vi "2017 Washer Backsplash Tester Main.vi"() -> ()   [LabVIEW 2016]
uses:
  controls/states.ctl
  controls/Stop Button.ctl
  controls/Test Results.ctl
  controls/Error_Command.ctl
  C:/Program Files (x86)/National Instruments/LabVIEW 2016/examples/Design Patterns/Queued Message Handler/support/QMH Fundamentals - Message Cluster.ctl
  C:/Automation/DLLs/PC Dot Net/GeaCommunication.dll
  Common/LabVIEW GEA2 Toolkit/LabVIEW_GEA2_Toolkit.lvlibp
panel:
  out "Test Results out":T1
  in  "Stop Button":T2
  out "State":T3
  in  "Barcode Scan":string
  out "Error Out":errorcluster
  in  "Error In":errorcluster
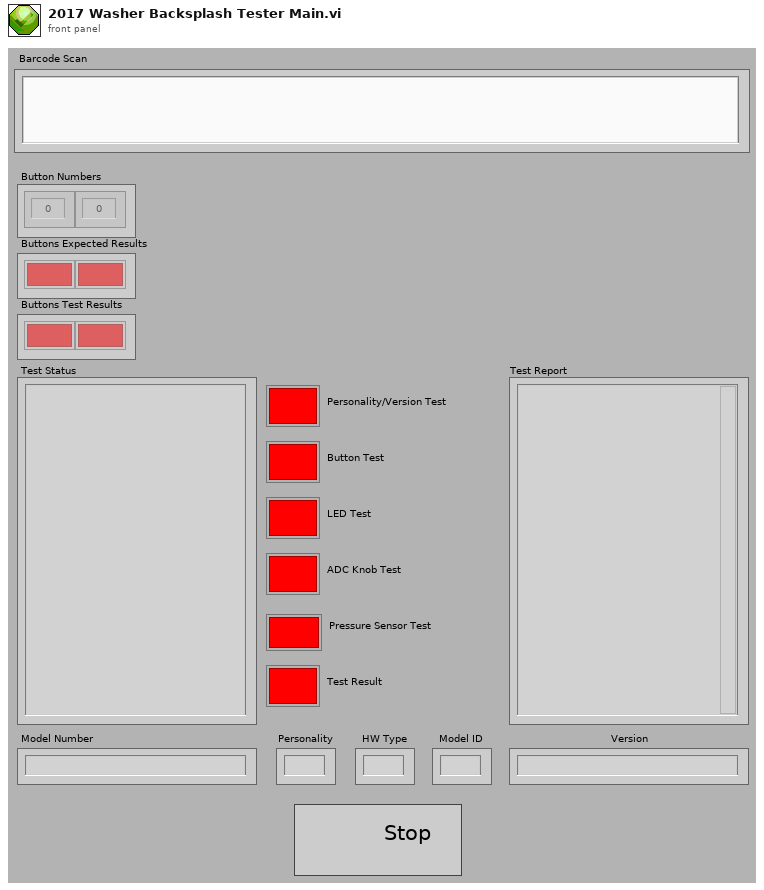
[diagram p1: front panel]
types:
  T1 = cluster{"Test Status":string, "Personality/Version Test ":bool, "Test Report":string, "Model Number":string, "Button Numbers":i32[], "Buttons Test Results":bool[], "Buttons Expected Results":bool[], "Model ID":string, "Personality":string, "HW Type":string, "Version":string, "Button Test":bool, "LED Test":bool, "ADC Knob Test":bool, "Pressure Sensor Test":bool, "Test Result":bool}
  T2 = typedef "Stop Button.ctl" = bool
  T3 = typedef "states.ctl" = enum16{"Wait for Barcode Scan", "Confirm Board Setup", "Initialization", "Perosnality Test", "Button Test", "LED Test", "ADC Knob Test", "Pressure Sensor Test", "Test Complete", "Log Results", "Re-Init Test", "Shutdown"}
  T4 = typedef "QMH Fundamentals - Message Cluster.ctl" = cluster{"Message":string, "Message Data":variant}
  T5 = typedef "Error_Command.ctl" = enum16{"Initialize", "Handle Errors", "Report Errors"}
  T6 = typedef "Test Results.ctl" = cluster{"Test Status":string, "Personality/Version Test ":bool, "Test Report":string, "Model Number":string, "Button Numbers":i32[], "Buttons Test Results":bool[], "Buttons Expected Results":bool[], "Model ID":string, "Personality":string, "HW Type":string, "Version":string, "Button Test":bool, "LED Test":bool, "ADC Knob Test":bool, "Pressure Sensor Test":bool, "Test Result":bool}
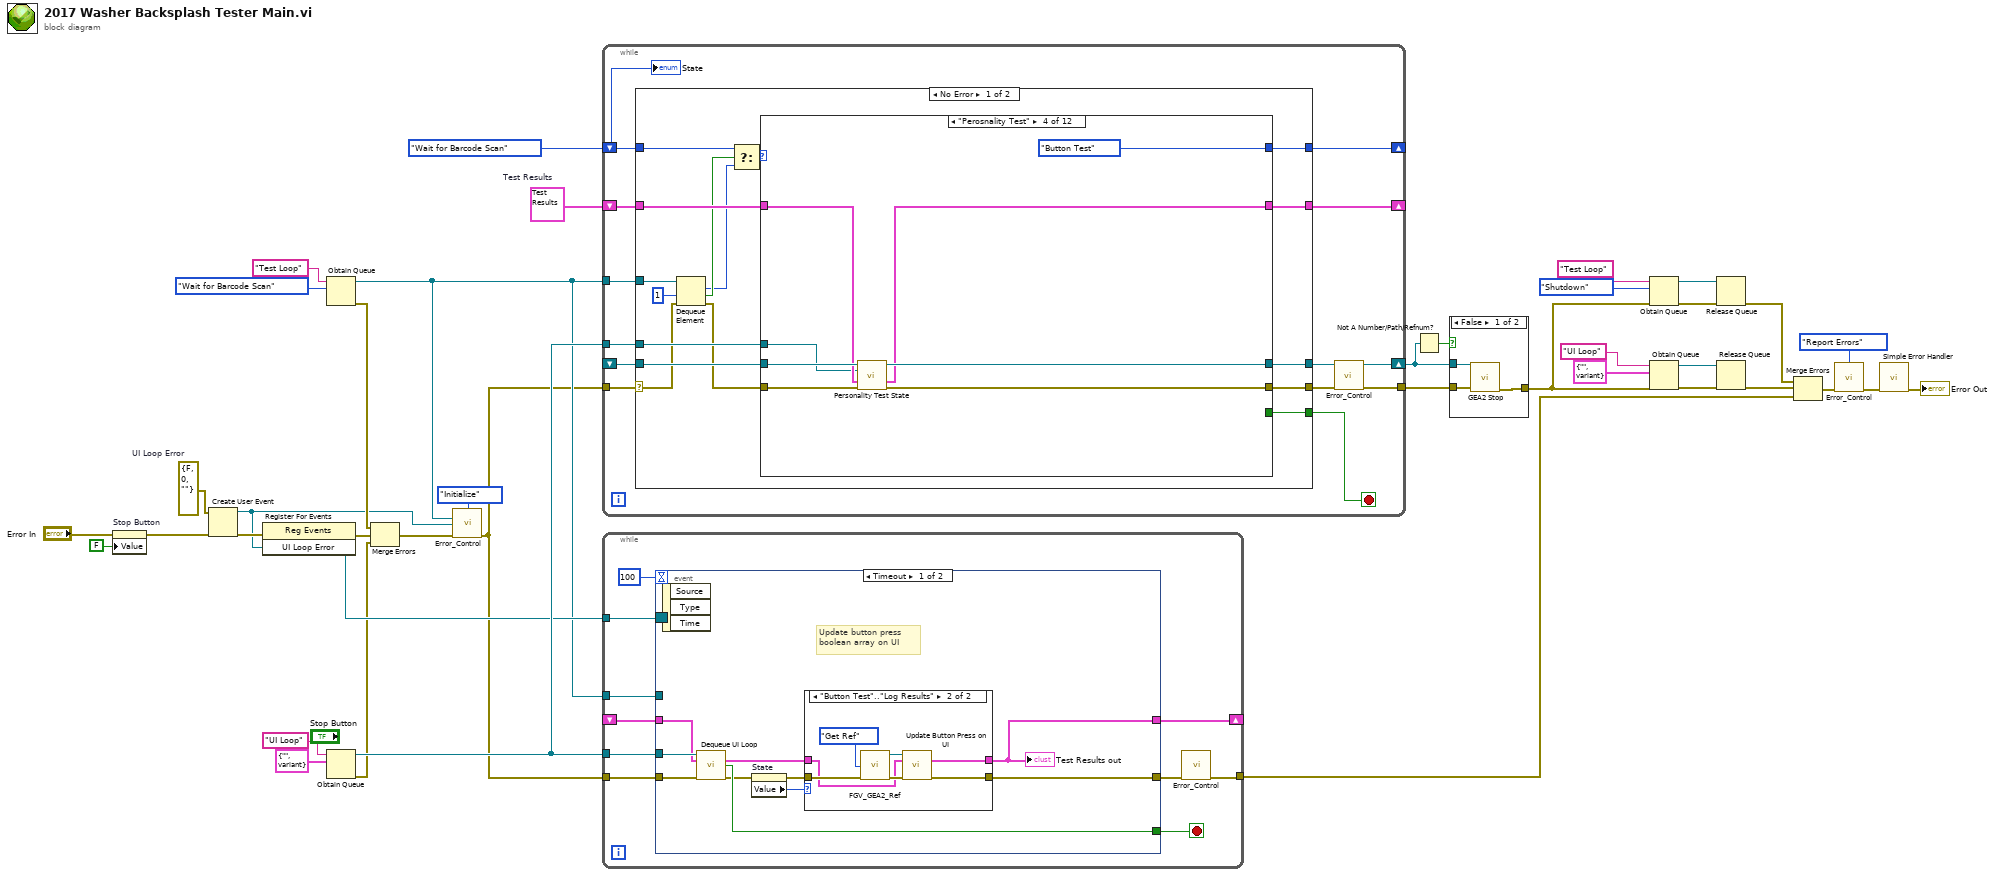
[diagram p0: block diagram]
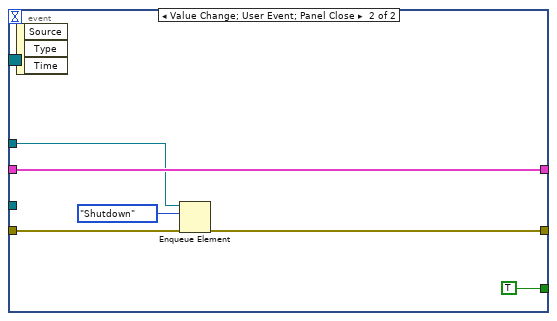
[diagram p4: hidden frame]
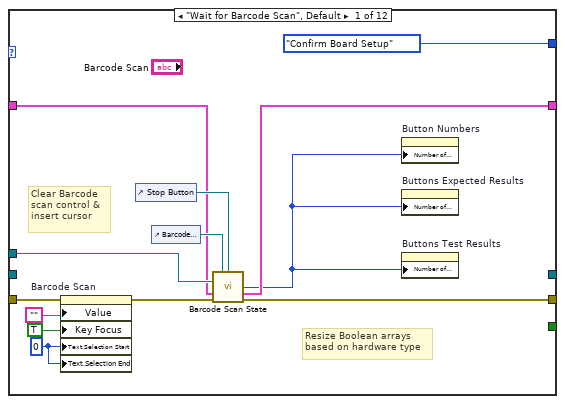
[diagram p5: hidden frame]
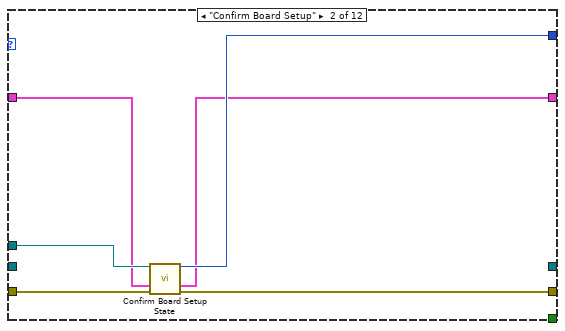
[diagram p6: hidden frame]
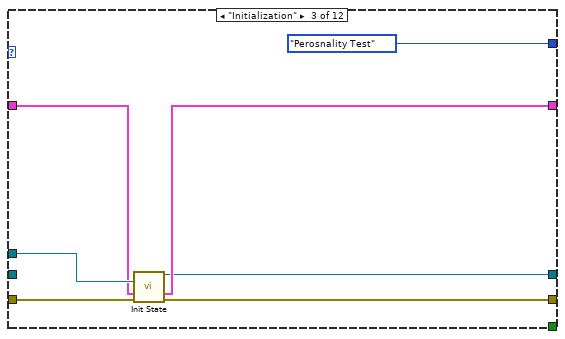
[diagram p7: hidden frame]
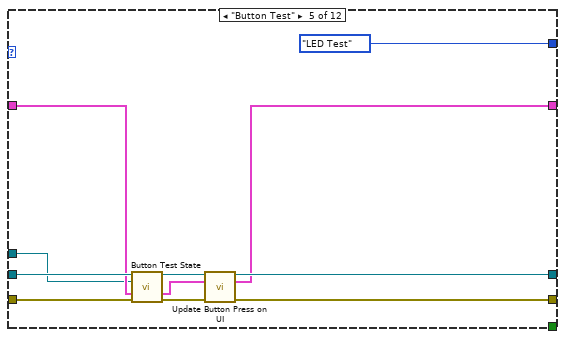
[diagram p8: hidden frame]
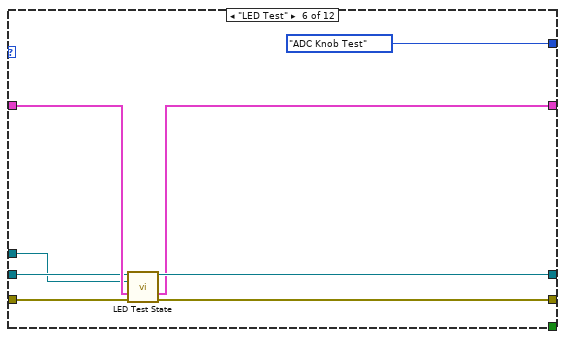
[diagram p9: hidden frame]
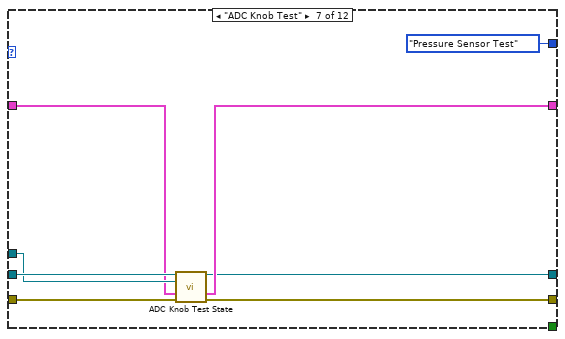
[diagram p10: hidden frame]
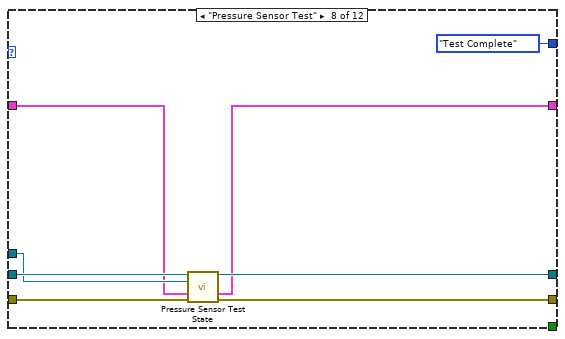
[diagram p11: hidden frame]
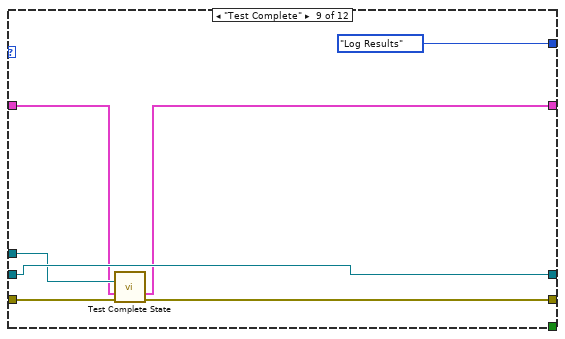
[diagram p12: hidden frame]
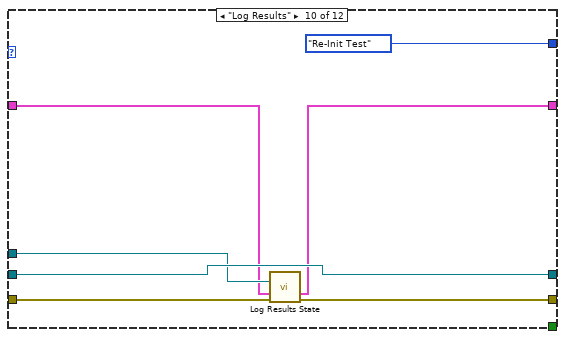
[diagram p13: hidden frame]
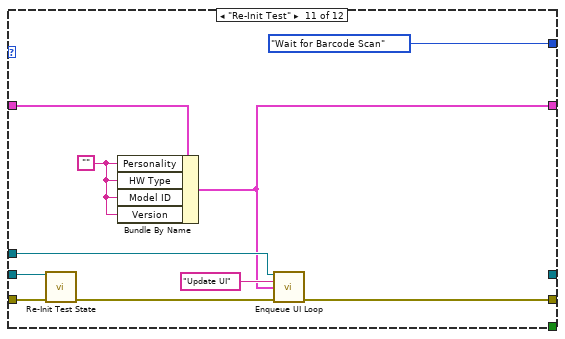
[diagram p14: hidden frame]
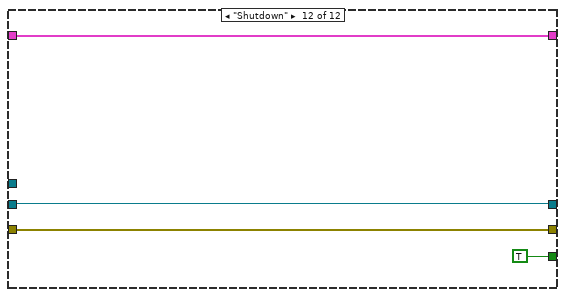
[diagram p15: hidden frame]
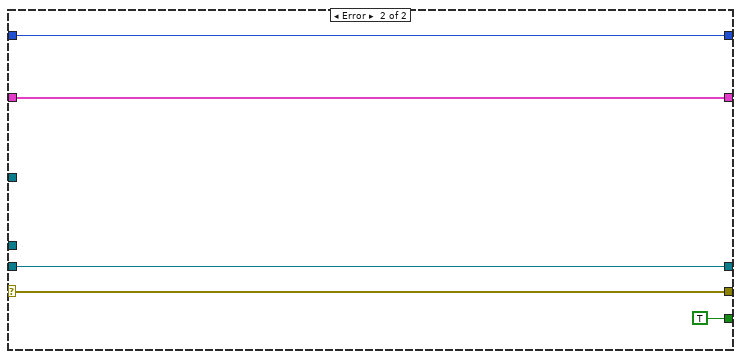
[diagram p16: hidden frame]
diagram:
  w14 = errorcluster {"status"=FALSE, "code"=0, "source"=""}  # UI Loop Error
  w39 = T6 {"Test Status"="", "Personality/Version Test "=FALSE, "Test Report"="", "Model Number"="", "Button Numbers"=[], "Buttons Test Results"=[], "Buttons Expected Results"=[], "Model ID"="", "Personality"="", "HW Type"="", "Version"="", "Button Test"=FALSE, "LED Test"=FALSE, "ADC Knob Test"=FALSE, "Pressure Sensor Test"=FALSE, "Test Result"=FALSE}  # Test Results
  n1 = property on="Stop Button" class="Bool (strict)"(error in="Error In", "Value"=FALSE ("Stop Button")) -> (error out=w13:errorcluster)  [unwired: 1 in, 1 out]
  n2 = Create User Event(user event datatype=w14, error in=w13) -> (user event=w8:refnum<user-event>, error out=w15:errorcluster)
  n3 = register-events(error in=w15, w8) -> (reference out=w11:refnum<event-registration>, error out=w3:errorcluster)  [unwired: 1 in]
  n4 = Obtain Queue(name (unnamed)="Test Loop", element data type=states."Wait for Barcode Scan" ("Enum")) -> (queue out=w9:refnum<queue>, error out=w12:errorcluster)  [unwired: 3 in, 1 out]
  n5 = Obtain Queue(name (unnamed)="UI Loop", element data type=T4 {"Message"="", "Message Data"=variant} ("Message Cluster")) -> (queue out=w38:refnum<queue>, error out=w2:errorcluster)  [unwired: 3 in, 1 out]
  n6 = Merge Errors(w12, w3, w2) -> (w10:errorcluster)
  n7 = call "Error_Control.vi"("Command (Handle Errors)"=Error_Command."Initialize", "Test Loop"=w9, "UI Loop Error"=w8, "Error In"=w10) -> ("Error Out"=w7:errorcluster)  [unwired: 11 in]
  n8 = while {
    shift-right: [w51] -> _
    shift-left: w39 -> [w52]
    shift-right: [w50] -> _
    shift-left: states."Wait for Barcode Scan" ("Enum") -> [w46]
    tunnel: [w42] -> w33
    shift-right: [w49] -> w27
    shift-left: _ -> [w48]
    tunnel: w38 -> [w47]
    tunnel: w9 -> [w45]
    tunnel: w7 -> [w41]
    stop <- w44 stop-if-true
    n9 = case shown="No Error" w41 {
      selector: w41 -> [w54 w169]
      tunnel: w46 -> [w58 w168]
      tunnel: w52 -> [w68 w167]
      tunnel: [w67 w167] -> w51
      tunnel: [w66 w168] -> w50
      tunnel: [w65 w169] -> w43
      tunnel: [w64 w170] -> w49
      tunnel: w48 -> [w63 w170]
      tunnel: w47 -> [w62 _]
      tunnel: w45 -> [w61 _]
      tunnel: [w56 TRUE] -> w44
      frame No Error {
        n10 = Dequeue Element(queue=w61, timeout in ms (-1)=1, error in (no error)=w54) -> (element=w57:T3, timed out?=w59:bool, error out=w53:errorcluster)  [unwired: 1 out]
        n11 = Select(t=w58, s=w59, f=w57) -> (s? t:f=w60:T3)
        n12 = case shown="\"Perosnality Test\"" w60 {
          tunnel: w68 -> [w74 w83 w88 w100 w111 w120 w124 w131 w140 w147 w155 w165]
          tunnel: [w73 w82 w92 w96 w104 w115 w123 w130 w138 w146 w154 w165] -> w67
          tunnel: [states."Confirm Board Setup" ("Enum") w87 states."Perosnality Test" ("Enum") states."Button Test" ("Enum") states."LED Test" ("Enum") states."ADC Knob Test" ("Enum") states."Pressure Sensor Test" ("Enum") states."Test Complete" ("Enum") states."Log Results" ("Enum") states."Re-Init Test" ("Enum") states."Wait for Barcode Scan" ("Enum") _] -> w66
          tunnel: w53 -> [w80 w86 w94 w99 w110 w118 w128 w136 w143 w145 w159 w164]
          tunnel: [w70 w85 w93 w97 w108 w116 w127 w134 w139 w149 w153 w164] -> w65
          tunnel: [_ _ w91 w101 w105 w121 w122 w133 w144 w150 _ w163] -> w64
          tunnel: w63 -> [_ _ _ w102 w112 w119 w126 w135 w144 w150 w160 w163]
          tunnel: w62 -> [w77 w84 w89 w98 w103 w117 w125 w132 w142 w148 w157 _]
          tunnel: [_ _ _ _ _ _ _ _ _ _ _ TRUE] -> w56
          frame "Wait for Barcode Scan", Default {
            w71 = u32 0 ("Text.Selection:Start")
            # "Clear Barcode\nscan control &\ninsert cursor"
            # "Resize Boolean arrays\nbased on hardware type"
            n13 = property on="Barcode Scan" class="Str"(error in=w80, "Value"="", "Key Focus"=TRUE, "Text.Selection Start"=w71, "Text.Selection End"=w71) -> (error out=w79:errorcluster)  [unwired: 1 in, 1 out]
            n14 = control-ref of="Stop Button"() -> (w75:refnum<vi>)
            n15 = control-ref of="Barcode Scan"() -> (w76:refnum<vi>)
            n16 = call "Barcode Scan State.vi"("Barcode Scan Refnum"=w76, "Stop Button Ref"=w75, "Queue in"=w77, "Test Results"=w74, "error in (no error)"=w79) -> ("Number of Buttons"=w69:u32, "Test Results Out"=w73:T6, "error out"=w70:errorcluster)  [unwired: 8 in]
            n17 = property on="Button Numbers" class="Arr (strict)"("Number of Columns"=w69) -> ()  [unwired: 2 in, 2 out]
            n18 = property on="Buttons Expected Results" class="Arr (strict)"("Number of Columns"=w69) -> ()  [unwired: 2 in, 2 out]
            n19 = property on="Buttons Test Results" class="Arr (strict)"("Number of Columns"=w69) -> ()  [unwired: 2 in, 2 out]
          }
          frame "Confirm Board Setup" {
            n20 = call "Confirm Board Setup State.vi"("Queue in"=w84, "Test Results in"=w83, "error in (no error)"=w86) -> ("State"=w87:T3, "Test Results out"=w82:T6, "error out"=w85:errorcluster)  [unwired: 10 in]
          }
          frame "Initialization" {
            n21 = call "Init State.vi"("Queue in"=w89, "Test Results in"=w88, "error in (no error)"=w94) -> (".NET Refnum out"=w91:refnum<k24>, "Test Results out"=w92:T6, "error out"=w93:errorcluster)  [unwired: 10 in]
          }
          frame "Perosnality Test" {
            n22 = call "Personality Test State.vi"("GEA2 Reference Out in"=w102, "Queue in"=w98, "Test Results in"=w100, "error in (no error)"=w99) -> (".NET Refnum out"=w101:refnum<k24>, "Test Results out"=w96:T6, "error out"=w97:errorcluster)  [unwired: 9 in]
          }
          frame "Button Test" {
            n23 = call "Button Test State.vi"("GEA2 Reference Out in"=w112, "Queue in"=w103, "Test Results in"=w111, "error in (no error)"=w110) -> (".NET Refnum out"=w106:refnum<k24>, "Test Results out"=w107:T6, "error out"=w109:errorcluster)  [unwired: 9 in]
            n24 = call "Update Button Press on UI.vi"("GEA2 Reference In"=w106, "Test Results in"=w107, "error in (no error)"=w109) -> ("GEA2 Reference Out"=w105:refnum<k24>, "Test Results out"=w104:T6, "error out"=w108:errorcluster)  [unwired: 10 in]
          }
          frame "LED Test" {
            n25 = call "LED Test State.vi"("GEA2 Reference Out"=w119, "Queue in"=w117, "Test Results in"=w120, "error in (no error)"=w118) -> (".NET Refnum out"=w121:refnum<k24>, "Test Results out"=w115:T6, "error out"=w116:errorcluster)  [unwired: 9 in]
          }
          frame "ADC Knob Test" {
            n26 = call "ADC Knob Test State.vi"("GEA2 Reference Out"=w126, "Queue in"=w125, "Test Results in"=w124, "error in (no error)"=w128) -> (".NET Refnum out"=w122:refnum<k24>, "Test Results out"=w123:T6, "error out"=w127:errorcluster)  [unwired: 9 in]
          }
          frame "Pressure Sensor Test" {
            n27 = call "Pressure Sensor Test State.vi"("GEA2 Reference Out"=w135, "Queue in"=w132, "Test Results in"=w131, "error in (no error)"=w136) -> (".NET Refnum out"=w133:refnum<k24>, "Test Results out"=w130:T6, "error out"=w134:errorcluster)  [unwired: 9 in]
          }
          frame "Test Complete" {
            n28 = call "Test Complete State.vi"("Queue in"=w142, "Test Results in"=w140, "Error In"=w143) -> ("Test Results out"=w138:T6, "Error Out"=w139:errorcluster)  [unwired: 11 in]
          }
          frame "Log Results" {
            n29 = call "Log Results State.vi"("Queue in"=w148, "Test Results in"=w147, "error in (no error)"=w145) -> ("Test Results out"=w146:T6, "error out"=w149:errorcluster)  [unwired: 11 in]
          }
          frame "Re-Init Test" {
            w152 = ""
            n30 = call "Re-Init Test State.vi"(".NET Refnum in"=w160, "error in (no error)"=w159) -> ("error out"=w156:errorcluster)  [unwired: 13 in]
            n31 = Bundle By Name(cluster=w155, "Personality"=w152, "HW Type"=w152, "Model ID"=w152, "Version"=w152) -> (w154:T6)
            n32 = call "Enqueue UI Loop.vi"("UI Que In"=w157, "Message"="Update UI", "Test Results"=w154, "error in (no error)"=w156) -> ("error out"=w153:errorcluster)  [unwired: 10 in, 1 out]
          }
          frame "Shutdown" {
          }
        }
      }
      frame Error {
      }
    }
    n33 = call "Error_Control.vi"("Error In"=w43) -> ("Error Out"=w42:errorcluster)  [unwired: 14 in]
    "State" <- w46
  }
  n34 = while {
    tunnel: w38 -> [w180]
    tunnel: [w173] -> w32
    shift-right: [w176] -> _
    shift-left: _ -> [w177]
    tunnel: w9 -> [w175]
    tunnel: w11 -> [w172]
    tunnel: w7 -> [w171]
    stop <- w178 stop-if-true
    n35 = event shown="[0] Timeout" {
      selector: w172 -> [_ _]
      dyn-events: _ -> [_ _]
      timeout: 100 -> [_ _]
      tunnel: w180 -> [w190 _]
      tunnel: [w189 TRUE ("Stop Button")] -> w178
      tunnel: [w188 w203] -> w174
      tunnel: w177 -> [w184 w204]
      tunnel: [w181 w204] -> w176
      tunnel: w175 -> [_ w202]
      tunnel: w171 -> [w182 w200]
      event Timeout {
        # "Update button press\nboolean array on UI"
        n36 = event-data() -> ()  [unwired: 1 in, 3 out]
        n37 = call "Dequeue UI Loop.vi"("Queue In"=w190, "Test Results In"=w184, "error in (no error)"=w182) -> ("Test Results out"=w183:T6, "Stop Button"=w189:bool, "error out"=w187:errorcluster)  [unwired: 10 in]
        n38 = property on="State" class="Enum (strict)"(error in=w187) -> (error out=w186:errorcluster, "Value"=w185:T3)  [unwired: 1 in, 1 out]
        n39 = case shown="\"Button Test\"..\"Log Results\"" w185 {
          tunnel: w186 -> [w192 w197]
          tunnel: [w192 w195] -> w188
          tunnel: w183 -> [w191 w194]
          tunnel: [w191 w193] -> w181
          frame Default {
          }
          frame "Button Test".."Log Results" {
            n40 = call "FGV_GEA2_Ref.vi"("Action"=enum16{"Set Ref", "Get Ref"}."Get Ref", "Error In"=w197) -> ("GEA2 Reference Out"=w198:refnum<k24>, "Error Out"=w196:errorcluster)  [unwired: 12 in]
            n41 = call "Update Button Press on UI.vi"("GEA2 Reference In"=w198, "Test Results in"=w194, "error in (no error)"=w196) -> ("Test Results out"=w193:T6, "error out"=w195:errorcluster)  [unwired: 10 in, 1 out]
          }
        }
        "Test Results out" <- w181
      }
      event Value Change; User Event; Panel Close {
        n42 = event-data() -> ()  [unwired: 1 in, 3 out]
        n43 = Enqueue Element(queue=w202, element=states."Shutdown" ("Enum"), error in (no error)=w200) -> (error out=w203:errorcluster)  [unwired: 1 in, 2 out]
      }
    }
    n44 = call "Error_Control.vi"("Error In"=w174) -> ("Error Out"=w173:errorcluster)  [unwired: 14 in]
  }
  n45 = Not A Number/Path/Refnum?(number/path/refnum=w27) -> (NaN/Path/Refnum?=w26:bool)
  n46 = case shown="False" w26 {
    tunnel: w33 -> [w208 w209]
    tunnel: [w207 w209] -> w18
    tunnel: w27 -> [w206 _]
    frame False {
      n47 = call "GEA2 Stop.vi"("GEA2 Reference In"=w206, "Error In"=w208) -> ("Error Out"=w207:errorcluster)  [unwired: 13 in]
    }
    frame True {
    }
  }
  n48 = Obtain Queue(name (unnamed)="Test Loop", element data type=states."Shutdown" ("Enum"), error in (no error)=w18) -> (queue out=w25:refnum<queue>, error out=w20:errorcluster)  [unwired: 2 in, 1 out]
  n49 = Obtain Queue(name (unnamed)="UI Loop", element data type=T4 {"Message"="", "Message Data"=variant} ("Message Cluster"), error in (no error)=w18) -> (queue out=w35:refnum<queue>, error out=w36:errorcluster)  [unwired: 2 in, 1 out]
  n50 = Release Queue(queue=w25, error in (no error)=w20) -> (error out=w19:errorcluster)  [unwired: 1 in, 2 out]
  n51 = Release Queue(queue=w35, error in (no error)=w36) -> (error out=w34:errorcluster)  [unwired: 1 in, 2 out]
  n52 = Merge Errors(w19, w34, w32) -> (w24:errorcluster)
  n53 = call "Error_Control.vi"("Command (Handle Errors)"=Error_Command."Report Errors", "Error In"=w24) -> ("Error Out"=w23:errorcluster)  [unwired: 13 in]
  n54 = call <vilib>:"Simple Error Handler.vi"("error in (no error)"=w23) -> ("error out"=→"Error Out":errorcluster)  [unwired: 4 in, 4 out]
